vi "Bear_simulator.vi"(10 "Angle 2":dbl[](array[numeric])=[0.0, -11.3, -11.2, -1.8, 6.3, -2.65, -30.4, -30.15, -27.15, -20.7, 0.0, 1.0, 19.9, 4.8, 6.0, 11.9, 19.9, 35.0, 34.5, 42.1, 41.9, 35.55, 90.0, 52.0, 0.0], 11 "Angle 1":dbl[](array[numeric])=[90.0, 88.6, 86.8, 84.0, 71.2, 60.15, 63.5, 54.4, 53.3, 57.1, 46.0, 39.6, 27.0, 37.0, 32.1, 27.85, 27.0, 23.6, 26.2, 21.58, 24.1, 28.3, 24.0, 53.8, 90.0]) -> (3 "3D Picture":refnum<vi>(3d-picture))   [LabVIEW 2024]
uses:
  <vilib>/Analysis/Matrix/Datatypes/RealMatrix.ctl
  <vilib>/Utility/miscctls.llb/LVRGBAColorTypeDef.ctl
  <vilib>/Utility/miscctls.llb/LV3DPointTypeDef.ctl
  <vilib>/Analysis/baseanly.llb/Real A x B.vi
  <vilib>/Analysis/Matrix/NI_Matrix.lvlib
  <vilib>/Analysis/NI_AALBase.lvlib
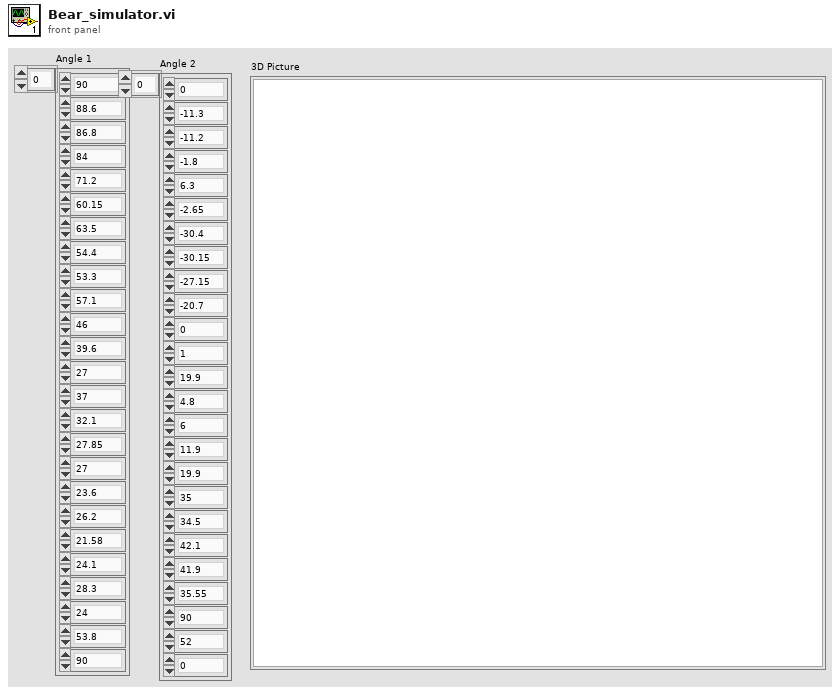
[diagram p1: front panel]
types:
  T1 = typedef "LV3DPointTypeDef.ctl" = cluster{"X":sgl, "Y":sgl, "Z":sgl}
  T2 = enum16{"None", "Spherical", "Flying", "Oriented"}
  T3 = typedef "LVRGBAColorTypeDef.ctl" = cluster{"Red":sgl, "Green":sgl, "Blue":sgl, "Alpha":sgl}
  T4 = typedef "NI_Matrix.lvlib/RealMatrix.ctl" = dbl[][]
  T5 = cluster{"Line width":sgl, "Line Color":u32, "Axes?":bool}
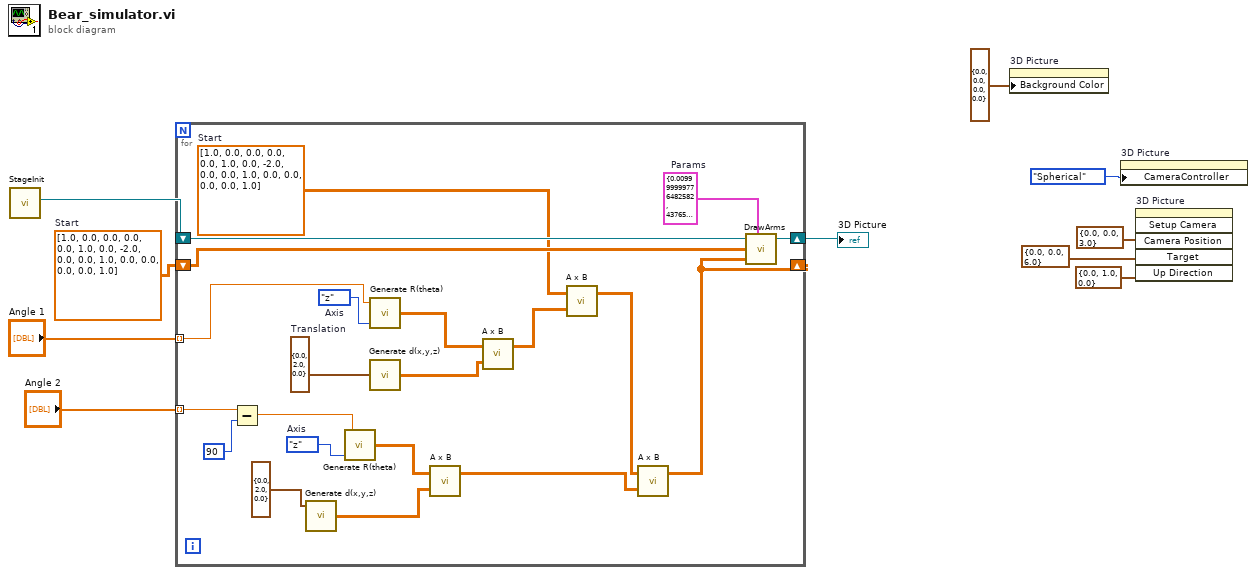
[diagram p0: block diagram]
diagram:
  w8 = T4 [[1.0, 0.0, 0.0, 0.0], [0.0, 1.0, 0.0, -2.0], [0.0, 0.0, 1.0, 0.0], [0.0, 0.0, 0.0, 1.0]]  # Start
  n1 = call <userlib>:"StageInit.vi"() -> ("Stage out"=w10:refnum<vi>)  [unwired: 4 in, 1 out]
  n2 = for {
    shift-right: [w21] -> w9
    shift-left: w10 -> [w22]
    shift-right: [w20] -> _
    shift-left: w8 -> [w19]
    tunnel: "Angle 1" -> [w16] mode=indexing
    tunnel: "Angle 2" -> [w11] mode=indexing
    w27 = enum16{"x", "y", "z"}."z"  # Axis
    w30 = cluster{"X":dbl, "Y":dbl, "Z":dbl} {"X"=0.0, "Y"=2.0, "Z"=0.0}  # Translation
    w31 = enum16{"x", "y", "z"}."z"  # Axis
    w14 = T4 [[1.0, 0.0, 0.0, 0.0], [0.0, 1.0, 0.0, -2.0], [0.0, 0.0, 1.0, 0.0], [0.0, 0.0, 0.0, 1.0]]  # Start
    w24 = T5 {"Line width"=0.01, "Line Color"=4376575, "Axes?"=FALSE}  # Params
    n3 = Subtract(x=w11, y=90) -> (x-y=w13:dbl)
    n4 = call <userlib>:"Generate d(x,y,z).vi"("Translation"=cluster{"X":dbl, "Y":dbl, "Z":dbl} {"X"=0.0, "Y"=2.0, "Z"=0.0}) -> ("Transformation Matrix"=w26:T4)  [unwired: 2 in]
    n5 = call <userlib>:"Generate R(theta).vi"("Axis"=w27, "Angle (degrees)"=w13) -> ("Transformation Matrix"=w25:T4)  [unwired: 1 in]
    n6 = call <userlib>:"Generate R(theta).vi"("Axis"=w31, "Angle (degrees)"=w16) -> ("Transformation Matrix"=w28:T4)  [unwired: 1 in]
    n7 = call <userlib>:"Generate d(x,y,z).vi"("Translation"=w30) -> ("Transformation Matrix"=w29:T4)  [unwired: 2 in]
    n8 = call-poly <vilib>:"A x B.vi"("B"=w26, "A"=w25) -> ("A x B"=w18:T4)  [unwired: 1 out]
    n9 = call-poly <vilib>:"A x B.vi"("B"=w29, "A"=w28) -> ("A x B"=w15:T4)  [unwired: 1 out]
    n10 = call-poly <vilib>:"A x B.vi"("B"=w15, "A"=w14) -> ("A x B"=w17:T4)  [unwired: 1 out]
    n11 = call-poly <vilib>:"A x B.vi"("B"=w18, "A"=w17) -> ("A x B"=w20:T4)  [unwired: 1 out]
    n12 = call <userlib>:"DrawArms.vi"("Stage in"=w22, "Params"=w24, "Start"=w19, "End"=w20) -> ("Stage out"=w21:refnum<vi>)  [unwired: 2 in, 1 out]
  }
  "3D Picture" <- w9
  n13 = property on="3D Picture" class="SceneGraphDisp (strict)"("Background Color"=T3 {"Red"=0.0, "Green"=0.0, "Blue"=0.0, "Alpha"=0.0}) -> ()  [unwired: 2 in, 2 out]
  n14 = property on="3D Picture" class="SceneGraphDisp (strict)"("CameraController"=T2."Spherical" ("Camera Controller:Type")) -> ()  [unwired: 2 in, 2 out]
  n15 = invoke on="3D Picture" class="SceneGraphDisp (strict)" method="Setup Camera"("Camera Position"=T1 {"X"=0.0, "Y"=0.0, "Z"=6.0}, "Target"=T1 {"X"=0.0, "Y"=0.0, "Z"=3.0}, "Up Direction"=T1 {"X"=0.0, "Y"=1.0, "Z"=0.0}) -> ()  [unwired: 3 in, 6 out]
